vi "take_mag_data.vi"(0 "magnetometer in":refnum<class "magnetometer.lvclass">, 1 "sampling info":cluster{"Fs":dbl, "#s":dbl}, 5 "restart averaging":bool, 7 "averaging parameters":T1={"averaging mode"=enum."No averaging", "weighting mode"=enum."Exponential", "number of averages"=10} {"number of averages" min=1}, 11 "error in (no error)":errorcluster) -> (4 "magnetometer out":refnum<class "magnetometer.lvclass">, 6 "mag 1 data":cluster{"f0":dbl, "df":dbl, "magnitude":dbl[]}, 8 "mag 2 data":cluster{"f0":dbl, "df":dbl, "magnitude":dbl[]}, 10 "difference":cluster{"f0":dbl, "df":dbl, "magnitude":dbl[]}, 15 "error out":errorcluster)   [LabVIEW 2015, in "magnetometer.lvclass"]
uses:
  magnetometer.lvclass
  <vilib>/Analysis/4window.llb/windowTd.ctl
  <vilib>/DAQmx/read.llb/DAQmx Read (Analog Wfm 1Chan NSamp).vi
  <vilib>/DAQmx/miscellaneous.llb/DAQmx Fill In Error Info.vi
  <vilib>/measure/maspectr.llb/FFT Power Spectrum and PSD for 1 Chan.vi
  <vilib>/measure/NI_MAPro.lvlib
  <vilib>/Analysis/NI_AALPro.lvlib
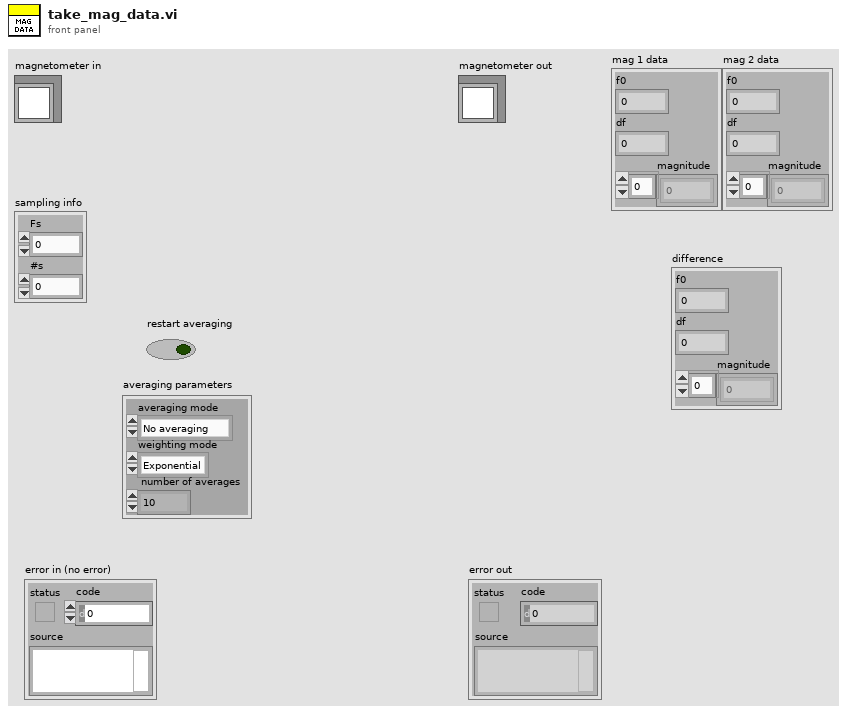
[diagram p1: front panel]
types:
  T1 = cluster{"averaging mode":enum16{"No averaging", "Vector averaging", "RMS averaging", "Peak hold"}, "weighting mode":enum16{"Linear", "Exponential"}, "number of averages":u32}
  T2 = typedef "NI_AALPro.lvlib/windowTd.ctl" = u32
  T3 = cluster{"input 1 task out":refnum<k21>, "input 2 task out":refnum<k21>}
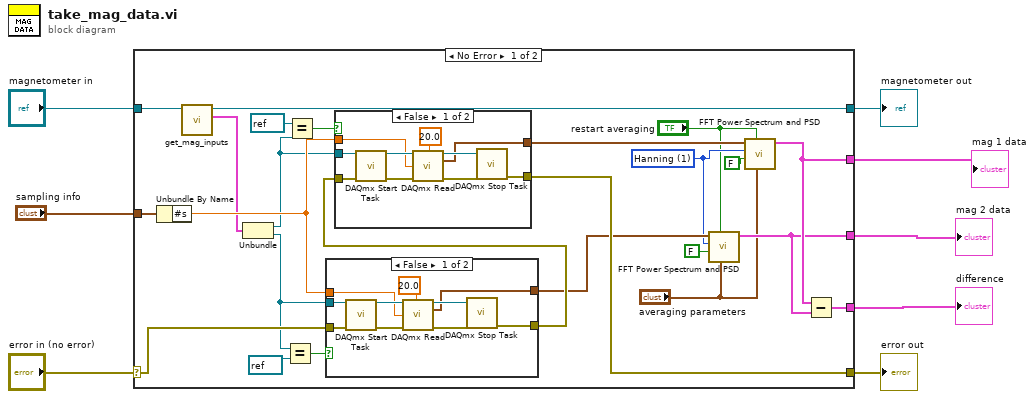
[diagram p0: block diagram]
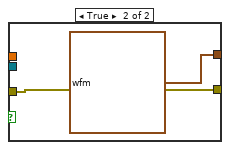
[diagram p2: hidden frame]
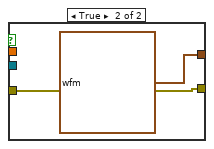
[diagram p3: hidden frame]
diagram:
  n1 = case shown="No Error" "error in (no error)" {
    selector: "error in (no error)" -> [w27 w58]
    tunnel: [w25 w58] -> w7
    tunnel: [w29 w57] -> w5
    tunnel: "magnetometer in" -> [w30 w57]
    tunnel: "sampling info" -> [w32 _]
    tunnel: [w15 _] -> w3
    tunnel: [w13 _] -> w2
    tunnel: [w18 _] -> w1
    frame No Error {
      w11 = T2 1 items=["Rectangle"=0, "Hanning"=1, "Hamming"=2, "Blackman-Harris"=3, "Exact Blackman"=4, "Blackman"=5, "Flat Top"=6, "4 Term B-Harris "=7, "7 Term B-Harris"=8, "Low Sidelobe"=9, "Blackman Nuttall"=11, "Triangle"=30, "Bartlett-Hanning"=31, "Bohman"=32, "Parzen"=33, "Welch"=34, "Kaiser"=60, "Dolph-Chebyshev"=61, "Gaussian"=62] ("window")
      n2 = Unbundle By Name(w32) -> ("#s"=w31:dbl)
      n3 = call-dynamic "get_mag_inputs.vi"("magnetometer in"=w30) -> ("mag inputs"=w28:T3, "magnetometer out"=w29:refnum<class "magnetometer.lvclass">)  [unwired: 8 in, 1 out]
      n4 = Unbundle(w28) -> ("input 1 task out"=w24:refnum<k21>, "input 2 task out"=w19:refnum<k21>)
      n5 = Equal?(x=w19, y=refnum<k21> refnum ("x")) -> (x = y?=w21:bool)
      n6 = Equal?(x=refnum<k21> refnum, y=w24) -> (x = y?=w23:bool)
      n7 = case shown="False" w21 {
        tunnel: w19 -> [w37 _]
        tunnel: w31 -> [w36 _]
        tunnel: [w35 waveform(dbl) {"t0"=timestamp(0 s since 1904-01-01), "dt"=1.0, "Y"=[]} ("data")] -> w14
        tunnel: w27 -> [w34 w44]
        tunnel: [w33 w44] -> w26
        frame False {
          n8 = call <vilib>:"DAQmx Start Task.vi"("task/channels in"=w37, "error in"=w34) -> ("task out"=w41:refnum<k21>, "error out"=w40:errorcluster)  [unwired: 12 in]
          n9 = call-poly <vilib>:"DAQmx Read.vi"("task/channels in"=w41, "number of samples per channel"=w36, "timeout"=20.0, "error in"=w40) -> ("task out"=w39:refnum<k21>, "data"=w35:waveform(dbl), "error out"=w38:errorcluster)  [unwired: 9 in]
          n10 = call <vilib>:"DAQmx Stop Task.vi"("task/channels in"=w39, "error in"=w38) -> ("error out"=w33:errorcluster)  [unwired: 12 in, 1 out]
        }
        frame True {
        }
      }
      n11 = case shown="False" w23 {
        tunnel: w24 -> [w49 _]
        tunnel: w31 -> [w48 _]
        tunnel: [w47 waveform(dbl) {"t0"=timestamp(0 s since 1904-01-01), "dt"=1.0, "Y"=[]} ("data")] -> w16
        tunnel: w26 -> [w46 w56]
        tunnel: [w45 w56] -> w25
        frame False {
          n12 = call <vilib>:"DAQmx Start Task.vi"("task/channels in"=w49, "error in"=w46) -> ("task out"=w53:refnum<k21>, "error out"=w52:errorcluster)  [unwired: 12 in]
          n13 = call-poly <vilib>:"DAQmx Read.vi"("task/channels in"=w53, "number of samples per channel"=w48, "timeout"=20.0, "error in"=w52) -> ("task out"=w51:refnum<k21>, "data"=w47:waveform(dbl), "error out"=w50:errorcluster)  [unwired: 9 in]
          n14 = call <vilib>:"DAQmx Stop Task.vi"("task/channels in"=w51, "error in"=w50) -> ("error out"=w45:errorcluster)  [unwired: 12 in, 1 out]
        }
        frame True {
        }
      }
      n15 = call-poly <vilib>:"FFT Power Spectrum and PSD.vi"("averaging parameters"="averaging parameters", "restart averaging (F)"="restart averaging", "dB On (F)"=FALSE, "window"=w11, "time signal"=w14) -> ("Power Spectrum / PSD"=w13:cluster{"f0":dbl, "df":dbl, "magnitude":dbl[]})  [unwired: 3 in, 3 out]
      n16 = call-poly <vilib>:"FFT Power Spectrum and PSD.vi"("averaging parameters"="averaging parameters", "restart averaging (F)"="restart averaging", "dB On (F)"=FALSE, "window"=w11, "time signal"=w16) -> ("Power Spectrum / PSD"=w15:cluster{"f0":dbl, "df":dbl, "magnitude":dbl[]})  [unwired: 3 in, 3 out]
      n17 = Subtract(x=w15, y=w13) -> (x-y=w18:cluster{"f0":dbl, "df":dbl, "magnitude":dbl[]})
    }
    frame Error {
    }
  }
  "error out" <- w7
  "magnetometer out" <- w5
  "mag 1 data" <- w3
  "mag 2 data" <- w2
  "difference" <- w1
